vi "To String.vi"(8 "error in (no error)":errorcluster, 11 "Double Float in":refnum<class "Abs_Time 1D.lvclass">) -> (0 "error out":errorcluster, 2 "String":string, 3 "Double Float out":refnum<class "Abs_Time 1D.lvclass">)   [LabVIEW 2021, in "Abs_Time 1D.lvclass"]
uses:
  Abs_Time 1D.lvclass
  C:/TSA/LV_Abstract/Source/Abs_Types/Numeric 1D/Abs_Numeric_1D.lvclass
  Numeric 1D/Abs_Numeric_1D.lvclass/Abs_Numeric_1D.ctl
  Abs_Time 1D.lvclass/Abs_Time 1D.ctl
  Numeric 1D/Properties/Read Units.vi
  Properties/Read UTC Time For String Format.vi
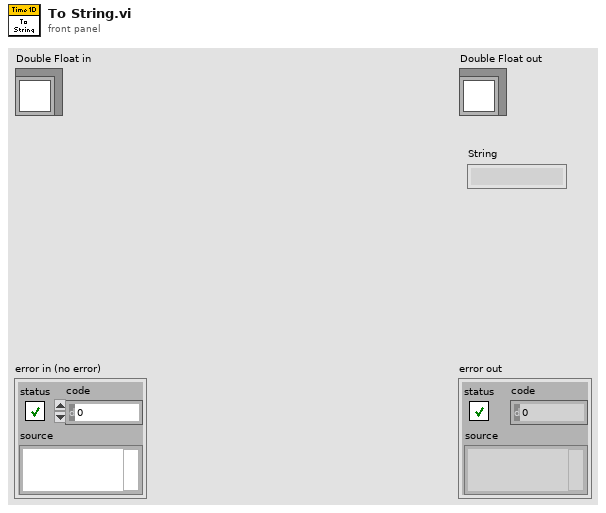
[diagram p1: front panel]
types:
  T1 = typedef "Abs_Time 1D.lvclass/Type.ctl" = timestamp[]
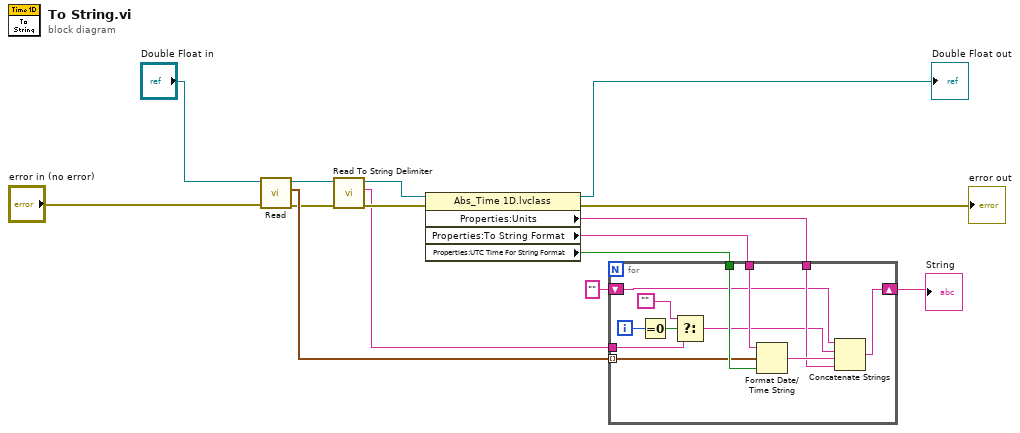
[diagram p0: block diagram]
diagram:
  n1 = call-dynamic "Read.vi"("error in (no error)"="error in (no error)", "Double Float.lvclass_340760 in"="Double Float in") -> ("error out"=w6:errorcluster, "Value"=w8:T1, "Double Float.lvclass_340760 out"=w7:refnum<class "Abs_Time 1D.lvclass">)  [unwired: 7 in]
  n2 = call-dynamic "Read To String Delimiter.vi"("error in (no error)"=w6, "Abs_Array in"=w7) -> ("error out"=w5:errorcluster, "To String Delimiter"=w3:string, "Abs_Array out"=w4:refnum<class "Abs_Time 1D.lvclass">)  [unwired: 7 in]
  n3 = property class="Abs_Time 1D.lvclass"(reference=w4, error in=w5) -> (reference out=→"Double Float out":refnum<class "Abs_Time 1D.lvclass">, error out=→"error out":errorcluster, "Properties:Units"=w9:string, "Properties:To String Format"=w11:string, "Properties:UTC Time For String Format"=w10:bool)
  n4 = for {
    tunnel: w10 -> [w25]
    tunnel: w9 -> [w24]
    tunnel: w11 -> [w26]
    tunnel: w8 -> [w23] mode=indexing
    tunnel: w3 -> [w18]
    shift-right: [w17] -> w2
    shift-left: "" -> [w16]
    i -> [w22]
    n5 = Equal To 0?(x=w22) -> (x = 0?=w21:bool)
    n6 = Select(t="", s=w21, f=w18) -> (s? t:f=w19:string)
    n7 = Format Date/Time String(time format string (%c)=w26, seconds (now)=w23, UTC format=w25) -> (date/time string=w27:string)
    n8 = Concatenate Strings(w16, w19, w27, w24) -> (w17:string)
  }
  "String" <- w2
